vi "ziGetEventComplexData.vi"(8 "Error In":errorcluster, 10 "Sample In":T1, 11 "Handle In":T2 {"Handle" format="0x%08x"; "Conn" format="0x%08x"}) -> (0 "Error Out":errorcluster, 2 "Sample Out":T1, 3 "Handle Out":T2 {"Handle" format="0x%08x"; "Conn" format="0x%08x"})   [LabVIEW 2018, in "Zurich Instruments LabOne.lvlib"]
uses:
  Zurich Instruments LabOne.lvlib
  <instrlib>/Zurich Instruments LabOne/Private/ziLV64.framework
  ziTypeHandle.ctl
  ziTypeComplexDataTS.ctl
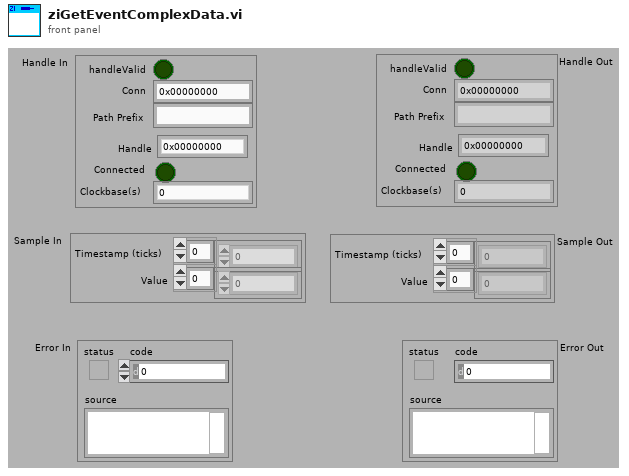
[diagram p1: front panel]
types:
  T1 = typedef "Zurich Instruments LabOne.lvlib/ziTypeComplexDataTS.ctl" = cluster{"Timestamp (ticks)":u64[], "Value":cdb[]}
  T2 = typedef "Zurich Instruments LabOne.lvlib/ziTypeHandle.ctl" = cluster{"handleValid":bool, "Conn":u64, "Path Prefix":string, "Handle":u64, "Connected":bool, "Clockbase(s)":dbl}
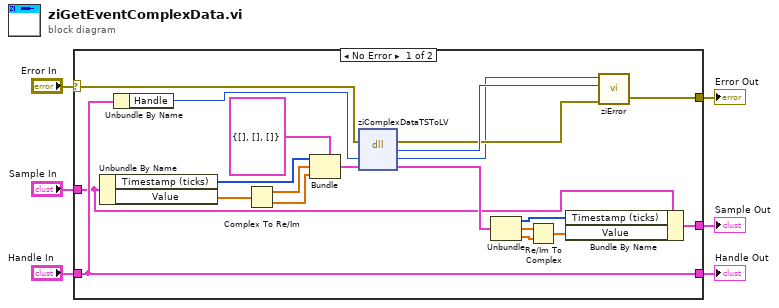
[diagram p0: block diagram]
diagram:
  n1 = case shown="No Error" "Error In" {
    selector: "Error In" -> [w26 w29]
    tunnel: "Handle In" -> [w21 w28]
    tunnel: [w21 w28] -> w5
    tunnel: "Sample In" -> [w10 w27]
    tunnel: [w25 w29] -> w3
    tunnel: [w7 w27] -> w1
    frame No Error {
      n2 = Unbundle By Name(w10) -> ("Timestamp (ticks)"=w18:u64[], "Value"=w19:cdb[])
      n3 = Unbundle By Name(w21) -> ("Handle"=w24:u64)
      n4 = Complex To Re/Im(x + iy=w19) -> (x=w16:dbl[], y=w15:dbl[])
      n5 = Bundle(cluster=cluster{u64[], dbl[], dbl[]} {[], [], []} ("input cluster"), w18, w16, w15) -> (w14:cluster{u64[], dbl[], dbl[]})
      n6 = dll-call lib="Applications/National Instruments/LabVIEW 2019 64-bit/instr.lib/Zurich Instruments LabOne/Private/ziLV*.*" fn="ziComplexDataTSToLV"(error in=w26, "ziEventBuffer"=w24, "DoubleSample"=w14) -> (error out=w22:errorcluster, "return type"=w23:u32, "ziEventBuffer"=w20:u64, "DoubleSample"=w13:cluster{u64[], dbl[], dbl[]})  [unwired: 2 in, 1 out]
      n7 = Unbundle(w13) -> (w9:u64[], w12:dbl[], w11:dbl[])
      n8 = Re/Im To Complex(1:w11, 2:w12) -> (0:w8:cdb[])
      n9 = Bundle By Name(cluster=w10, "Timestamp (ticks)"=w9, "Value"=w8) -> (w7:T1)
      n10 = call "ziError.vi"("Conn"=w20, "ziErrorCode"=w23, "Error In"=w22) -> ("Error Out"=w25:errorcluster)  [unwired: 2 in, 1 out]
    }
    frame Error {
    }
  }
  "Handle Out" <- w5
  "Sample Out" <- w1
  "Error Out" <- w3
